vi "CSTK_BuildApplication_Manager_setSetting.vi"(8 "Error in":errorcluster caption="错误输入", 10 "BuildApplication Selector":T1={"Package as a ZIP file?"=TRUE, "Rename EXE File Name?"=FALSE}) -> (0 "Error out":errorcluster caption="错误输出")   [LabVIEW 2015, in "CSTK_BuildApplication_Manager.lvlib"]
uses:
  CSTK_BuildApplication_Manager.lvlib
  CSTK_BuildApplication_Manager_selector.ctl
  <vilib>/addons/_JKI.lib/Serialization/JSON/JKI JSON Serialization.lvlib
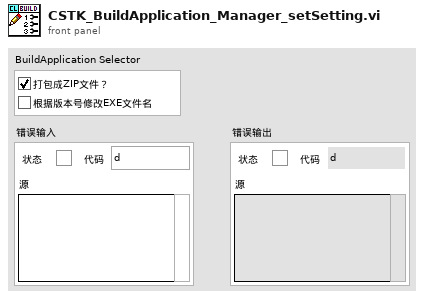
[diagram p1: front panel]
types:
  T1 = typedef "CSTK_BuildApplication_Manager.lvlib/CSTK_BuildApplication_Manager_selector.ctl" = cluster{"Package as a ZIP file?":bool, "Rename EXE File Name?":bool}
  T2 = enum16{"open", "replace", "create", "open or create", "replace or create", "replace or create with confirmation"}
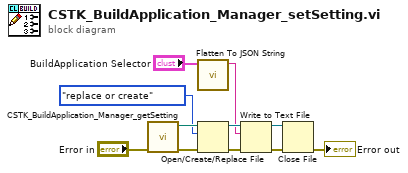
[diagram p0: block diagram]
diagram:
  n1 = call "CSTK_BuildApplication_Manager_getSetting.vi"("Error in"="Error in") -> ("Error out"=w9:errorcluster, "Setting path"=w11:path)  [unwired: 8 in, 1 out]
  n2 = call <vilib>:"Flatten To JSON String.vi"("Variant"="BuildApplication Selector") -> ("JSON String"=w3:string)  [unwired: 9 in, 1 out]
  n3 = Open/Create/Replace File(file path (use dialog)=w11, error in=w9, operation (0:open)=T2."replace or create" ("操作(0:open)")) -> (refnum out=w7:refnum<file>, error out=w8:errorcluster)  [unwired: 3 in, 1 out]
  n4 = Write to Text File(file (use dialog)=w7, text=w3, error in=w8) -> (refnum out=w6:refnum<file>, error out=w5:errorcluster)  [unwired: 1 in, 1 out]
  n5 = Close File(refnum=w6, error in=w5) -> (error out=→"Error out":errorcluster)  [unwired: 1 out]
